vi "NiFPGA Read - Boolean.vi"(8 "error in (no error)":errorcluster, 10 "Indicator":u32, 11 "Session":u32) -> (0 "error out":errorcluster, 1 "Boolean":bool, 3 "Session Out":u32)   [LabVIEW 2010, in "FPGA Interface Wrapper.lvlib"]
doc: "Reads a boolean value from a given indicator or control."
uses:
  <userlib>/_FPGA Interface Advanced Tools/FPGA Interface Wrapper/FPGA Interface Wrapper.lvlib
  NiFpga.dll
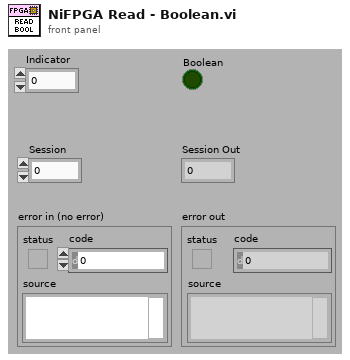
[diagram p1: front panel]
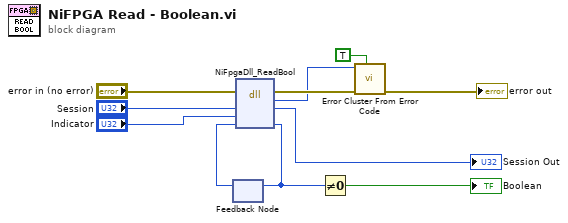
[diagram p0: block diagram]
diagram:
  n1 = feedback #1() -> (w1:u8)  [unwired: 1 in]
  n2 = dll-call lib="NiFpga.dll" fn="NiFpgaDll_ReadBool"(error in="error in (no error)", "Session"="Session", "Indicator"="Indicator", "Value"=w1) -> (error out=w5:errorcluster, "Status"=w4:i32, "Session"=→"Session Out":u32, "Value"=w2:u8)  [unwired: 3 in, 1 out]
  n3 = feedback-in #1(w2) -> ()
  n4 = Not Equal To 0?(x=w2) -> (x != 0?=→"Boolean":bool)
  n5 = call <vilib>:"Error Cluster From Error Code.vi"("show call chain? (False)"=TRUE, "error in (no error)"=w5, "error code (0)"=w4) -> ("error out"=→"error out":errorcluster)  [unwired: 6 in]
